vi "Historesis.vi"(2 "Reinitialize":bool, 3 "Input":i32) -> (0 "Same?":bool, 1 "Output":i32)   [LabVIEW 2012]
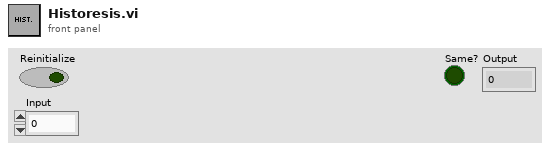
[diagram p1: front panel]
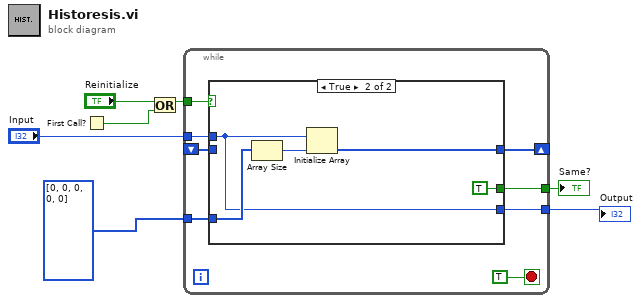
[diagram p0: block diagram]
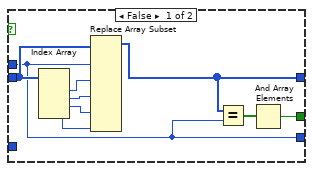
[diagram p2: hidden frame]
diagram:
  n1 = First Call?() -> (First Call?: T/F=w5:bool)
  n2 = Or(x="Reinitialize", y=w5) -> (x .or. y?=w6:bool)
  n3 = while {
    tunnel: w6 -> [w15]
    shift-right: [w12] -> _
    shift-left: _ -> [w13]
    tunnel: i32[] [0, 0, 0, 0, 0] -> [w11]
    tunnel: "Input" -> [w10]
    tunnel: [w9] -> w2
    tunnel: [w8] -> w1
    stop <- TRUE stop-if-true
    n4 = case shown="True" w15 {
      tunnel: w11 -> [_ w27]
      tunnel: w13 -> [w24 _]
      tunnel: [w19 w28] -> w12
      tunnel: w10 -> [w16 w25]
      tunnel: [w17 TRUE] -> w9
      tunnel: [w16 w25] -> w8
      frame False {
        n5 = Index Array(array=w24) -> (element #1=w23:i32, element #2=w22:i32, element #3=w21:i32, element #4=w20:i32)  [unwired: 4 in]
        n6 = Replace Array Subset(array=w24, new element #1=w16, new element #2=w23, new element #3=w22, new element #4=w21, new element #5=w20) -> (w19:i32[])  [unwired: 5 in]
        n7 = Equal?(x=w19, y=w16) -> (x = y?=w18:bool[])
        n8 = And Array Elements(Boolean array=w18) -> (logical AND=w17:bool)
      }
      frame True {
        n9 = Array Size(array=w27) -> (size(s)=w29:i32)
        n10 = Initialize Array(w25, w29) -> (w28:i32[])
      }
    }
  }
  "Same?" <- w2
  "Output" <- w1
